vi "test_stopIfTaskAlreadyStoppedShouldReturnNoError.vi"(11 "Test Case In":refnum<class "TaskControllerTests.lvclass">) -> (0 "error out":errorcluster, 3 "Test Case Out":refnum<class "TaskControllerTests.lvclass">)   [LabVIEW 2023, in "TaskControllerTests.lvclass"]
uses:
  TaskControllerTests.lvclass
  <vilib>/Astemes/LUnit/Test Case.lvclass/Test Case.ctl
  <vilib>/Astemes/LUnit/Core/LUnit Test Case/Private/Append Pass Result.vi
  <vilib>/Astemes/LUnit/Core/LUnit Test Case/Private/Append Fail Result.vi
  <vilib>/Astemes/LUnit/Core/LUnit Test Case/Private/Run In UI.vi
  <vilib>/Utility/error.llb/Clear Errors.vi
  TLC_Connect/source/LabVIEW/TaskMock/TaskMock.lvclass
  TLC_Connect/source/LabVIEW/TaskController/TaskController.lvclass
  <vilib>/Astemes/LUnit/Test Case.lvclass
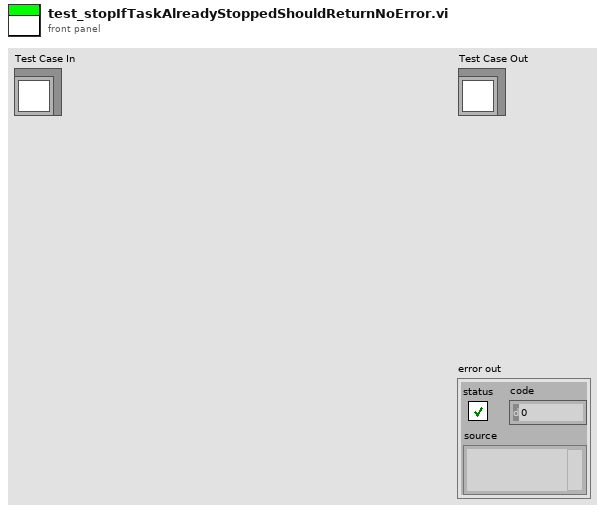
[diagram p1: front panel]
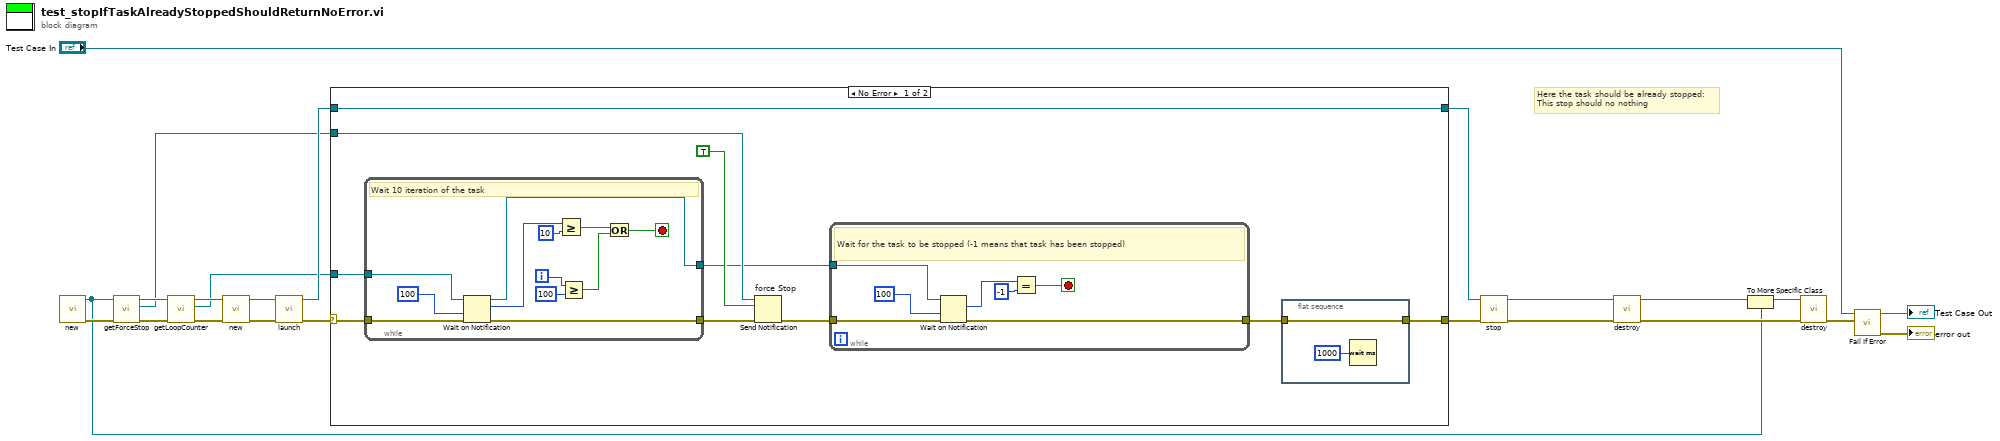
[diagram p0: block diagram]
diagram:
  # "Here the task should be already stopped:\nThis stop should no nothing"
  n1 = call "new.vi"() -> ("error out"=w9:errorcluster, "TaskMock out"=w2:refnum<class "TaskMock.lvclass">)  [unwired: 10 in]
  n2 = call "getForceStop.vi"("error in (no error)"=w9, "TaskMock in"=w2) -> ("error out"=w4:errorcluster, "forceStop"=w1:refnum<notifier>, "TaskMock out"=w3:refnum<class "TaskMock.lvclass">)  [unwired: 7 in]
  n3 = call "getLoopCounter.vi"("error in (no error)"=w4, "TaskMock in"=w3) -> ("error out"=w8:errorcluster, "loopCounter"=w15:refnum<notifier>, "TaskMock out"=w16:refnum<class "TaskMock.lvclass">)  [unwired: 7 in]
  n4 = call "new.vi"("error in (no error)"=w8, "task"=w16) -> ("error out"=w19:errorcluster, "TaskController out"=w20:refnum<class "TaskController.lvclass">)  [unwired: 8 in]
  n5 = call "launch.vi"("error in (no error)"=w19, "TaskController in"=w20) -> ("error out"=w17:errorcluster, "TaskController out"=w18:refnum<class "TaskController.lvclass">)  [unwired: 8 in]
  n6 = case shown="No Error" w17 {
    selector: w17 -> [w33 _]
    tunnel: w18 -> [w31 w55]
    tunnel: w15 -> [w32 _]
    tunnel: [w31 w55] -> w14
    tunnel: [w24 _] -> w13
    tunnel: w1 -> [w30 _]
    frame No Error {
      n7 = while {
        tunnel: w33 -> [w45]
        tunnel: w32 -> [w54]
        tunnel: [w44] -> w28
        tunnel: [w43] -> w26
        i -> [w50]
        stop <- w47 stop-if-true
        # "Wait 10 iteration of the task"
        n8 = Wait on Notification(notifier=w54, timeout in ms (-1)=100, error in (no error)=w45) -> (notifier out=w43:refnum<notifier>, notification=w52:i32, error out=w44:errorcluster)  [unwired: 1 in, 1 out]
        n9 = Greater Or Equal?(x=w52, y=10) -> (x >= y?=w48:bool)
        n10 = Greater Or Equal?(x=w50, y=100) -> (x >= y?=w46:bool)
        n11 = Or(x=w48, y=w46) -> (x .or. y?=w47:bool)
      }
      n12 = Send Notification "force Stop"(notification=TRUE, notifier=w30, error in (no error)=w28) -> (error out=w27:errorcluster)  [unwired: 1 out]
      n13 = while {
        tunnel: w27 -> [w39]
        tunnel: w26 -> [w42]
        tunnel: [w38] -> w25
        stop <- w36 stop-if-true
        # "Wait for the task to be stopped (-1 means that task has been stopped)"
        n14 = Wait on Notification(notifier=w42, timeout in ms (-1)=100, error in (no error)=w39) -> (notification=w40:i32, error out=w38:errorcluster)  [unwired: 1 in, 2 out]
        n15 = Equal?(x=w40, y=-1) -> (x = y?=w36:bool)
      }
      n16 = flat-sequence {
        tunnel: w25 -> [w34]
        tunnel: [w34] -> w24
        frame #0 {
          n17 = Wait (ms)(milliseconds to wait=u32 1000) -> ()  [unwired: 1 out]
        }
      }
    }
    frame Error {
    }
  }
  n18 = call "stop.vi"("error in (no error)"=w13, "TaskController in"=w14) -> ("error out"=w7:errorcluster, "TaskController out"=w6:refnum<class "TaskController.lvclass">)  [unwired: 8 in]
  n19 = call "destroy.vi"("error in (no error)"=w7, "TaskController in"=w6) -> ("error out"=w12:errorcluster, "task"=w11:refnum<class "ITask.lvclass">)  [unwired: 8 in]
  n20 = To More Specific Class(target class=w2, reference=w11) -> (specific class reference=w10:refnum<class "TaskMock.lvclass">)  [unwired: 1 in, 1 out]
  n21 = call "destroy.vi"("error in (no error)"=w12, "TaskMock in"=w10) -> ("error out"=w5:errorcluster)  [unwired: 9 in]
  n22 = call <vilib>:"Fail If Error.vi"("Assert error"=w5, "LUnit Test Case In"="Test Case In") -> ("error out"=→"error out":errorcluster, "LUnit Test Case Out"=→"Test Case Out":refnum<class "TaskControllerTests.lvclass">)  [unwired: 8 in]
